vi "Get all VIs in Project excluding Test Case VIs.vi"(8 "error in (no error)":errorcluster, 10 "Path":path, 11 "Coverage Analyzer in":refnum<class "Coverage Analyzer.lvclass">) -> (0 "error out":errorcluster, 2 "VIs":set{path}(c389), 3 "Coverage Analyzer out":refnum<class "Coverage Analyzer.lvclass">)   [LabVIEW 2020, in "Coverage Analyzer.lvclass"]
uses:
  Coverage Analyzer.lvclass
  2fa7b275-f75d-4bcf-8530-71b3ed265666.vi
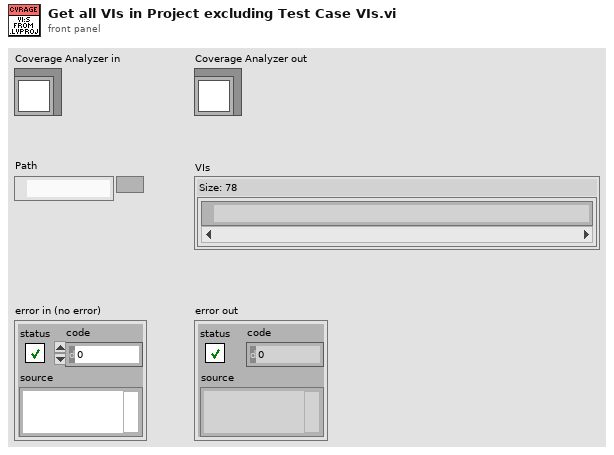
[diagram p1: front panel]
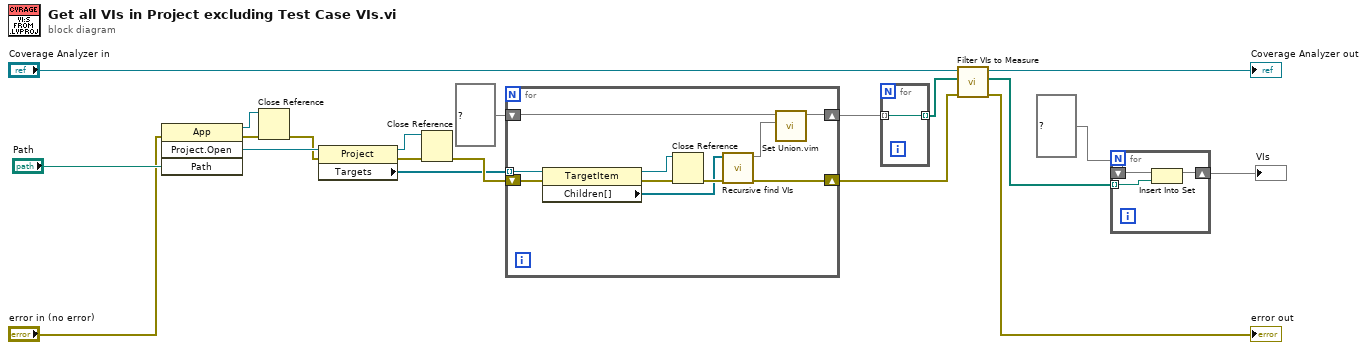
[diagram p0: block diagram]
diagram:
  n1 = invoke class="App" method="Project.Open"(error in="error in (no error)", "Path"="Path") -> (reference out=w12:refnum<vi>, error out=w17:errorcluster, "Project:Open"=w19:refnum<vi>)  [unwired: 2 in, 1 out]
  n2 = Close Reference(reference=w12, error in (no error)=w17) -> (error out=w13:errorcluster)
  n3 = property class="Project"(reference=w19, error in=w13) -> (reference out=w14:refnum<vi>, error out=w18:errorcluster, "Targets"=w1:refnum<vi>[])
  n4 = Close Reference(reference=w14, error in (no error)=w18) -> (error out=w15:errorcluster)
  n5 = for {
    tunnel: w1 -> [w30] mode=indexing
    shift-right: [w27] -> w8
    shift-left: w15 -> [w28]
    shift-right: [w23] -> w6
    shift-left: set{path} {} ("VIs") -> [w25]
    n6 = property class="TargetItem"(reference=w30, error in=w28) -> (reference out=w26:refnum<vi>, error out=w29:errorcluster, "Children[]"=w21:refnum<vi>[])
    n7 = Close Reference(reference=w26, error in (no error)=w29) -> (error out=w22:errorcluster)
    n8 = call "Recursive find VIs.vi"("error in (no error)"=w22, "Project Items"=w21) -> ("error out"=w27:errorcluster, "VIs"=w24:set{path})  [unwired: 8 in]
    n9 = call "Set Union.vim"("set 2"=w24, "set 1"=w25) -> ("union"=w23:set{path})  [unwired: 9 in]
  }
  n10 = for {
    tunnel: w6 -> [w31] mode=indexing
    tunnel: [w31] -> w5 mode=indexing
  }
  n11 = call "Filter VIs to Measure.vi"("error in (no error)"=w8, "VI Paths"=w5, "Coverage Analyzer in"="Coverage Analyzer in") -> ("error out"=→"error out":errorcluster, "Filtered VI Paths"=w2:path[], "Coverage Analyzer out"=→"Coverage Analyzer out":refnum<class "Coverage Analyzer.lvclass">)  [unwired: 6 in]
  n12 = for {
    shift-right: [w33] -> w3
    shift-left: set{path} {} ("VIs") -> [w34]
    tunnel: w2 -> [w32] mode=indexing
    n13 = Insert Into Set(10:w32, 11:w34) -> (3:w33:set{path})  [unwired: 1 out]
  }
  "VIs" <- w3
